vi "Start Y Tovey.vi"(8 "error in (no error)":errorcluster, 11 "Model in":refnum<class "Model.lvclass">) -> (0 "error out":errorcluster, 3 "Model out":refnum<class "Model.lvclass">)   [LabVIEW 2016, in "Model.lvclass"]
uses:
  Model.lvclass
  Model.lvclass/Model.ctl
  TEI-9150/Tovey 9150.lvclass
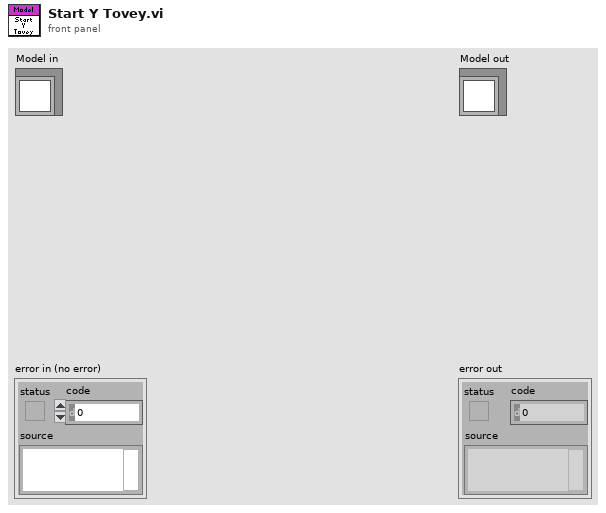
[diagram p1: front panel]
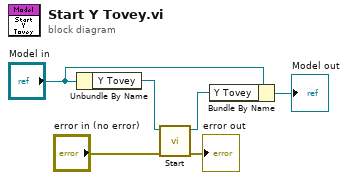
[diagram p0: block diagram]
diagram:
  n1 = Unbundle By Name("Model in") -> ("Y Tovey"=w4:refnum<class "Tovey 9150.lvclass">)
  n2 = call "Start.vi"("error in (no error)"="error in (no error)", "Tovey9150 in"=w4) -> ("error out"=→"error out":errorcluster, "Tovey9150 out"=w3:refnum<class "Tovey 9150.lvclass">)  [unwired: 8 in]
  n3 = Bundle By Name(cluster="Model in", "Y Tovey"=w3) -> (→"Model out":refnum<class "Model.lvclass">)
